vi "Set Text Definition.vi"(10 "Text Definition":T1, 11 "Text in":refnum<class "Text.lvclass">) -> (3 "Text out":refnum<class "Text.lvclass">)   [LabVIEW 2020, in "Conditu2.lvlib" / "Columns.lvlib" / "Text.lvclass"]
uses:
  Text.lvclass
  Definition.ctl
  Text.lvclass/Text.ctl
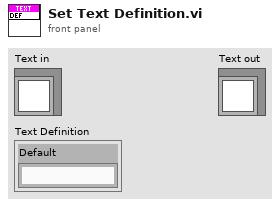
[diagram p1: front panel]
types:
  T1 = typedef "Conditu2.lvlib/Columns.lvlib/Text.lvclass/Definition.ctl" = cluster{"Default":string}
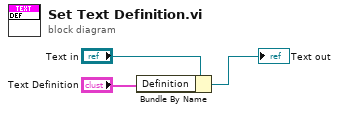
[diagram p0: block diagram]
diagram:
  n1 = Bundle By Name(cluster="Text in", "Definition"="Text Definition") -> (→"Text out":refnum<class "Text.lvclass">)
